vi "Optimize Pod Setpoints.vi"(7 "Current Pod Steering (deg)":cluster{"LF":dbl, "LB":dbl, "RF":dbl, "RB":dbl}, 10 "Initial Pod Setpoints (ft/s and deg)":T1) -> (2 "Optimized Pod Setpoints (ft/s and deg)":T1)   [LabVIEW 2020]
uses:
  ctl/Pod Setpoints.ctl
  <vilib>/Analysis/coordinate.llb/Wrap Angle.vi
  <vilib>/Analysis/coordinate.llb/Wrap Angle (scalar).vi
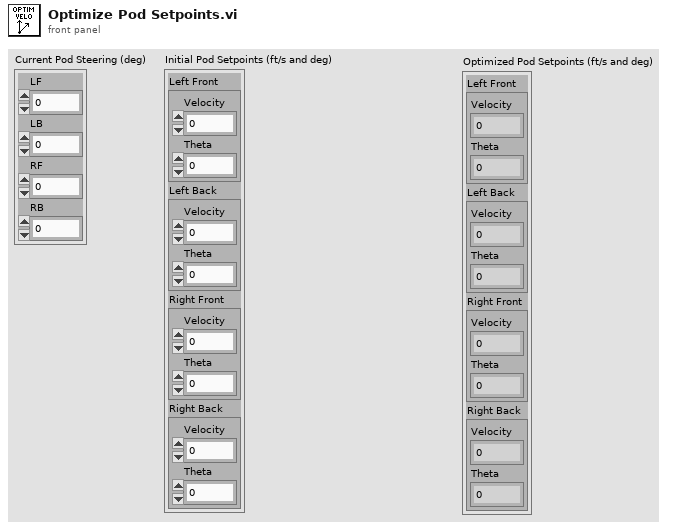
[diagram p1: front panel]
types:
  T1 = typedef "Pod Setpoints.ctl" = cluster{"Left Front":cluster{"Velocity":dbl, "Theta":dbl}, "Left Back":cluster{"Velocity":dbl, "Theta":dbl}, "Right Front":cluster{"Velocity":dbl, "Theta":dbl}, "Right Back":cluster{"Velocity":dbl, "Theta":dbl}}
  T2 = cluster{"[0]":cluster{"velocity":dbl, "travel angle":dbl}, "[1]":cluster{"velocity":dbl, "travel angle":dbl}, "[2]":cluster{"velocity":dbl, "travel angle":dbl}, "[3]":cluster{"velocity":dbl, "travel angle":dbl}}
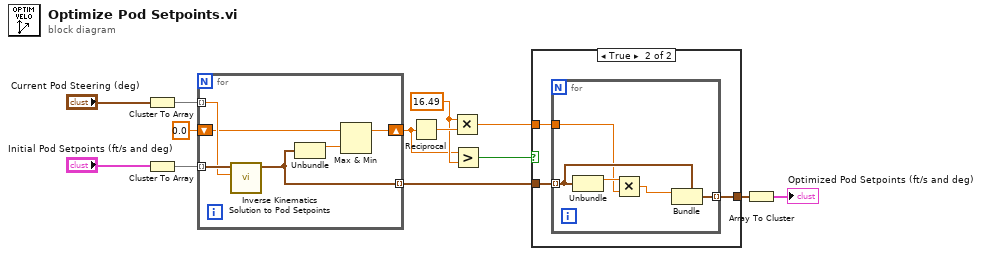
[diagram p0: block diagram]
diagram:
  w4 = 16.49 ("x")
  n1 = Cluster To Array(cluster="Current Pod Steering (deg)") -> (array=w10:dbl[])
  n2 = Cluster To Array(cluster="Initial Pod Setpoints (ft/s and deg)") -> (array=w13:cluster{"Velocity":dbl, "Theta":dbl}[])
  n3 = for {
    tunnel: w13 -> [w19] mode=indexing
    tunnel: w10 -> [w18] mode=indexing
    shift-right: [w14] -> w3
    shift-left: 0.0 -> [w15]
    tunnel: [w17] -> w8 mode=indexing
    n4 = call "Inverse Kinematics Solution to Pod Setpoints.vi"("actual theta"=w18, "v + target"=w19) -> ("new v + travel"=w17:cluster{"velocity":dbl, "travel angle":dbl})  [unwired: 9 in]
    n5 = Unbundle(w17) -> ("velocity"=w16:dbl)  [unwired: 1 out]
    n6 = Max & Min(x=w15, y=w16) -> (max(x,y)=w14:dbl)  [unwired: 1 out]
  }
  n7 = Reciprocal(x=w3) -> (1/x=w9:dbl)
  n8 = Multiply(x=w4, y=w9) -> (x*y=w7:dbl)
  n9 = Greater?(x=w3, y=w4) -> (0:w2:bool)
  n10 = case shown="True" w2 {
    tunnel: w8 -> [w20 w23]
    tunnel: w7 -> [_ w22]
    tunnel: [w20 w21] -> w6
    frame False {
    }
    frame True {
      n11 = for {
        tunnel: w23 -> [w27] mode=indexing
        tunnel: w22 -> [w25]
        tunnel: [w28] -> w21 mode=indexing
        n12 = Unbundle(w27) -> ("velocity"=w26:dbl)  [unwired: 1 out]
        n13 = Multiply(x=w26, y=w25) -> (x*y=w24:dbl)
        n14 = Bundle(cluster=w27, "velocity"=w24) -> (w28:cluster{"velocity":dbl, "travel angle":dbl})  [unwired: 1 in]
      }
    }
  }
  n15 = Array To Cluster(array=w6) -> (cluster=→"Optimized Pod Setpoints (ft/s and deg)":T2)
